vi "CLI Parameters--constant.vi"() -> (3 "CLI Parameters":T1[](array[typedef]))   [LabVIEW 2025]
doc: "This constant defines all Options of the g-secrets CLI interface. The parameters defined in this constant are used for parsing options and to generate the help message."
uses:
  <vilib>/Wiresmith Technology/G CLI/Argument Parser/Option Class/Option Configuration.ctl
  <vilib>/Wiresmith Technology/G CLI/Argument Parser/Option Class/Argument Type.ctl
  <vilib>/Wiresmith Technology/G CLI/Argument Parser/Option Class/Option.lvclass
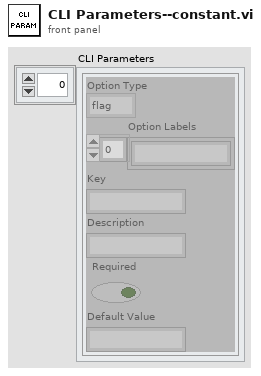
[diagram p1: front panel]
types:
  T1 = typedef "Option Parser.lvlib/Option.lvclass/Option Configuration.ctl" = cluster{"Option Type":T2, "Option Labels":string[], "Key":string, "Description":string, "Required":bool, "Default Value":string}
  T2 = typedef "Option Parser.lvlib/Option.lvclass/Argument Type.ctl" = enum16{"flag", "value"}
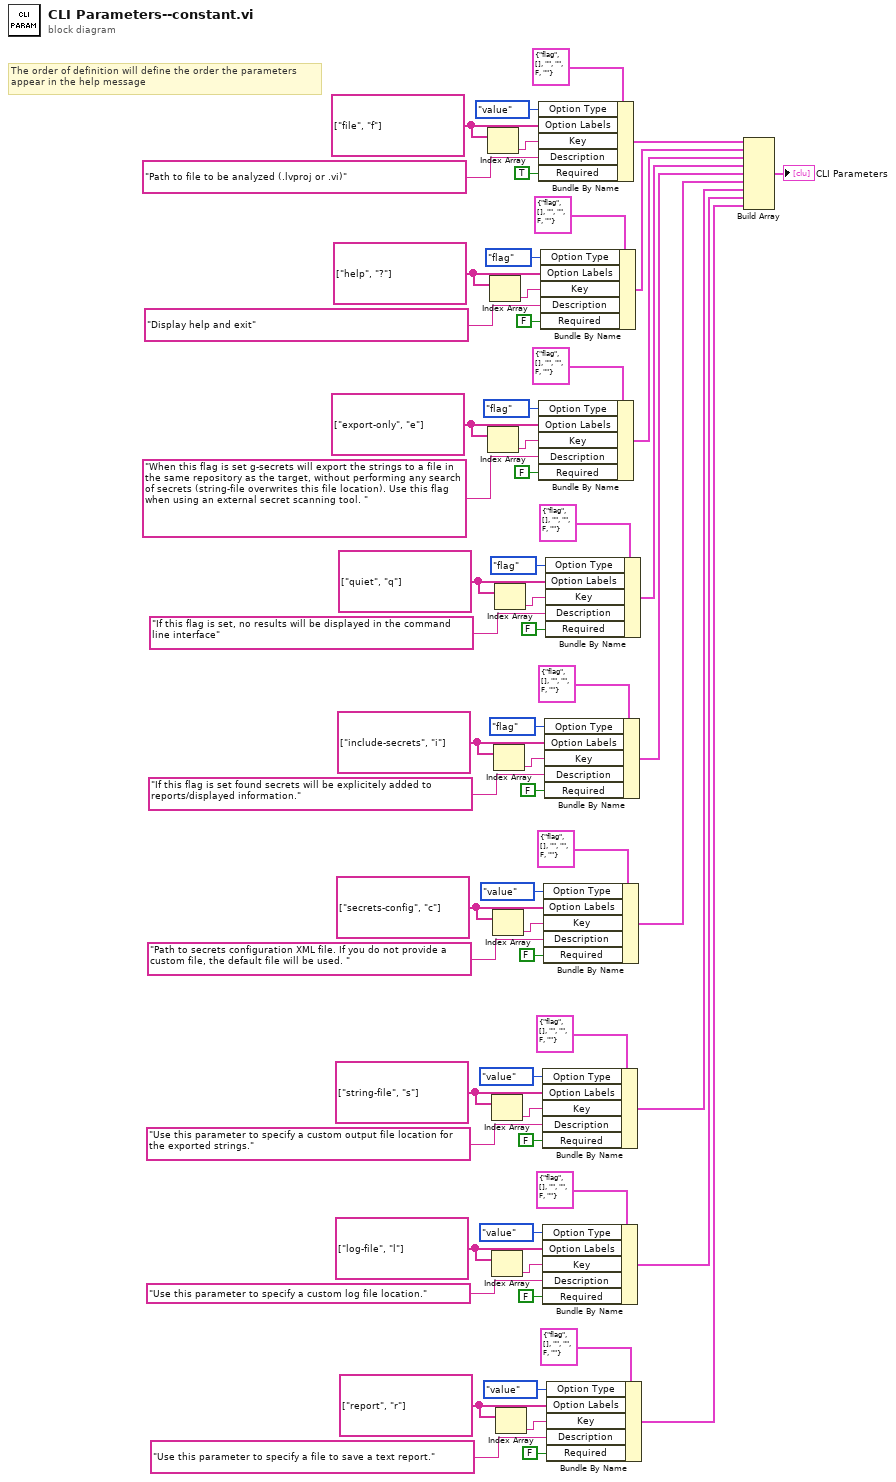
[diagram p0: block diagram]
diagram:
  w6 = string[] ["secrets-config", "c"] ("Option Labels")
  w21 = string[] ["file", "f"] ("Option Labels")
  w27 = string[] ["help", "?"] ("Option Labels")
  w33 = string[] ["include-secrets", "i"] ("Option Labels")
  w39 = string[] ["report", "r"] ("Option Labels")
  w45 = string[] ["quiet", "q"] ("Option Labels")
  w51 = string[] ["log-file", "l"] ("Option Labels")
  w57 = string[] ["string-file", "s"] ("Option Labels")
  w63 = string[] ["export-only", "e"] ("Option Labels")
  # "The order of definition will define the order the parameters\nappear in the help message"
  n1 = Index Array(array=w21) -> (element=w22:string)  [unwired: 1 in]
  n2 = Index Array(array=w63) -> (element=w64:string)  [unwired: 1 in]
  n3 = Index Array(array=w27) -> (element=w28:string)  [unwired: 1 in]
  n4 = Index Array(array=w57) -> (element=w58:string)  [unwired: 1 in]
  n5 = Index Array(array=w51) -> (element=w52:string)  [unwired: 1 in]
  n6 = Index Array(array=w6) -> (element=w7:string)  [unwired: 1 in]
  n7 = Index Array(array=w33) -> (element=w34:string)  [unwired: 1 in]
  n8 = Index Array(array=w45) -> (element=w46:string)  [unwired: 1 in]
  n9 = Index Array(array=w39) -> (element=w40:string)  [unwired: 1 in]
  n10 = Bundle By Name(cluster=T1 {"Option Type"=enum."flag", "Option Labels"=[], "Key"="", "Description"="", "Required"=FALSE, "Default Value"=""} ("Options"), "Option Type"=Argument_Type."value", "Option Labels"=w21, "Key"=w22, "Description"="Path to file to be analyzed (.lvproj or .vi)", "Required"=TRUE) -> (w16:T1)
  n11 = Bundle By Name(cluster=T1 {"Option Type"=enum."flag", "Option Labels"=[], "Key"="", "Description"="", "Required"=FALSE, "Default Value"=""} ("Options"), "Option Type"=Argument_Type."flag", "Option Labels"=w63, "Key"=w64, "Description"="When this flag is set g-secrets will export the strings to a file in the same repository as the target, without performing any search of secrets (string-file overwrites this file location). Use this flag when using an external secret scanning tool. ", "Required"=FALSE) -> (w14:T1)
  n12 = Bundle By Name(cluster=T1 {"Option Type"=enum."flag", "Option Labels"=[], "Key"="", "Description"="", "Required"=FALSE, "Default Value"=""} ("Options"), "Option Type"=Argument_Type."flag", "Option Labels"=w27, "Key"=w28, "Description"="Display help and exit", "Required"=FALSE) -> (w15:T1)
  n13 = Bundle By Name(cluster=T1 {"Option Type"=enum."flag", "Option Labels"=[], "Key"="", "Description"="", "Required"=FALSE, "Default Value"=""} ("Options"), "Option Type"=Argument_Type."value", "Option Labels"=w57, "Key"=w58, "Description"="Use this parameter to specify a custom output file location for the exported strings.", "Required"=FALSE) -> (w11:T1)
  n14 = Bundle By Name(cluster=T1 {"Option Type"=enum."flag", "Option Labels"=[], "Key"="", "Description"="", "Required"=FALSE, "Default Value"=""} ("Options"), "Option Type"=Argument_Type."value", "Option Labels"=w51, "Key"=w52, "Description"="Use this parameter to specify a custom log file location.", "Required"=FALSE) -> (w10:T1)
  n15 = Bundle By Name(cluster=T1 {"Option Type"=enum."flag", "Option Labels"=[], "Key"="", "Description"="", "Required"=FALSE, "Default Value"=""} ("Options"), "Option Type"=Argument_Type."value", "Option Labels"=w6, "Key"=w7, "Description"="Path to secrets configuration XML file. If you do not provide a custom file, the default file will be used. ", "Required"=FALSE) -> (w1:T1)
  n16 = Bundle By Name(cluster=T1 {"Option Type"=enum."flag", "Option Labels"=[], "Key"="", "Description"="", "Required"=FALSE, "Default Value"=""} ("Options"), "Option Type"=Argument_Type."flag", "Option Labels"=w33, "Key"=w34, "Description"="If this flag is set found secrets will be explicitely added to reports/displayed information.", "Required"=FALSE) -> (w12:T1)
  n17 = Bundle By Name(cluster=T1 {"Option Type"=enum."flag", "Option Labels"=[], "Key"="", "Description"="", "Required"=FALSE, "Default Value"=""} ("Options"), "Option Type"=Argument_Type."flag", "Option Labels"=w45, "Key"=w46, "Description"="If this flag is set, no results will be displayed in the command line interface", "Required"=FALSE) -> (w13:T1)
  n18 = Bundle By Name(cluster=T1 {"Option Type"=enum."flag", "Option Labels"=[], "Key"="", "Description"="", "Required"=FALSE, "Default Value"=""} ("Options"), "Option Type"=Argument_Type."value", "Option Labels"=w39, "Key"=w40, "Description"="Use this parameter to specify a file to save a text report.", "Required"=FALSE) -> (w9:T1)
  n19 = Build Array(w16, w15, w14, w13, w12, w1, w11, w10, w9) -> (→"CLI Parameters":T1[])
